vi "get path to lvdt presets.vi"(10 "product":string, 11 "paths.Base Path":path) -> (3 "path":path)   [LabVIEW 2018]
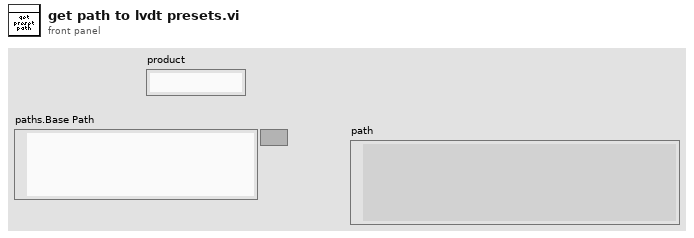
[diagram p1: front panel]
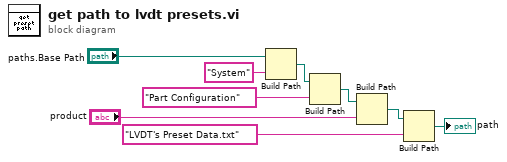
[diagram p0: block diagram]
diagram:
  n1 = Build Path(base path="paths.Base Path", name or relative path="System") -> (appended path=w4:path)
  n2 = Build Path(base path=w4, name or relative path="Part Configuration") -> (appended path=w5:path)
  n3 = Build Path(base path=w5, name or relative path="product") -> (appended path=w6:path)
  n4 = Build Path(base path=w6, name or relative path="LVDT's Preset Data.txt") -> (appended path=→"path":path)
